vi "Calculate_Deployment_LibInfo.vi"(8 "error in (no error)":errorcluster, 9 "main destination":path, 10 "destinations":refnum<class "AB_Destination.lvclass">[](array[class]), 11 "AB_EXE in":refnum<class "AB_EXE.lvclass">) -> (0 "error out":errorcluster, 2 "Lib Deployment Info":T1, 3 "AB_EXE out":refnum<class "AB_EXE.lvclass">)   [LabVIEW 2020, in "AB_EXE.lvclass"]
uses:
  <vilib>/AppBuilder/AB_Classes/EXE/AB_EXE.lvclass
  <vilib>/AppBuilder/AB_Classes/EXE/AB_EXE.lvclass/AB_EXE.ctl
  <vilib>/AppBuilder/AB_Classes/Build/AB_Build.lvclass
  <vilib>/AppBuilder/AB_Classes/Source/AB_Source.lvclass
  <vilib>/AppBuilder/AB_Classes/Destination/AB_Destination.lvclass
  <vilib>/AppBuilder/Engine/AB_Engine_RTDEP_Dep_Lib_Info.ctl
  <vilib>/AppBuilder/Engine/AB_Engine_RTDEP_LibDeploymentInfo.ctl
  <vilib>/Utility/lvfile.llb/NI_FileType.lvlib
  <vilib>/Utility/lvfile.llb/FT_FileTypes.ctl
  e:/builds/penguin/labview/branches/2020/dev/dist/vi.lib/AppBuilder/AB_Classes/Application/AB_Application.lvclass
  e:/builds/penguin/labview/branches/2020/dev/dist/vi.lib/AppBuilder/AB_Classes/TargetFile/AB_Targetfile.lvclass
  e:/builds/penguin/labview/branches/2020/dev/dist/vi.lib/AppBuilder/AB_Classes/Build/AB_Build.lvclass
  e:/builds/penguin/labview/branches/2020/dev/dist/vi.lib/AppBuilder/AB_Classes/EXE/AB_EXE.lvclass
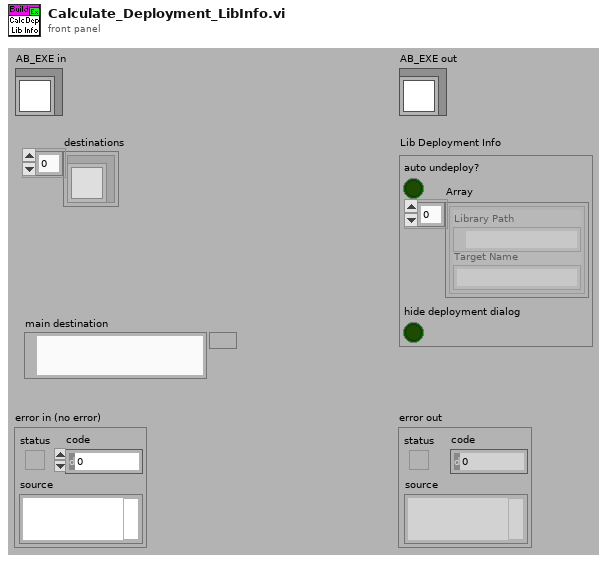
[diagram p1: front panel]
types:
  T1 = typedef "AB_Engine_RTDEP_LibDeploymentInfo.ctl" = cluster{"auto undeploy?":bool, "Array":T2[], "hide deployment dialog":bool}
  T2 = typedef "AB_Engine_RTDEP_Dep_Lib_Info.ctl" = cluster{"Library Path":path, "Target Name":string}
  T3 = typedef "NI_FileType.lvlib/FT_FileTypes.ctl" = enum32{"Invalid file/path", "Unknown type", "Instrument", "Control", "Polymorphic VI", "Project", "Library", "LVClass", "XControl", "XNode", "CIN", "Run-time menu", "Palette menu", "LLB", "Shortcut", "Directory", "Class Private Data Control", "Statechart", "MathScript .m file", "Ladder Diagram", "LVLibp"}
  T4 = typedef "AB_EXE_SharedVar_LibInfo.ctl" = cluster{"LibraryPath":path, "LibraryItemID":string, "target":string, "deploy":bool}
  T5 = typedef "AB_Source.ctl" = cluster{"path":path, "itemID":string, "parentIndex":i32, "sourceInclusion":T6, "destinationIndex":i32, "properties":T7[], "newName":string, "lvfile":bool, "valid":bool, "eng_inBuild":bool, "eng_isNonVILink":bool, "Amalgamation":bool, "Amalgamation Piece":bool, "eng_delimitedName":string, "preventRename":bool}
  T6 = typedef "AB_Source_Inclusion.ctl" = enum16{"IncludeIfReferenced", "Include", "Exclude", "TopLevel"}
  T7 = typedef "AB_Source_Properties.ctl" = cluster{"sourcePropertyType":T8, "value":variant}
  T8 = typedef "AB_Source_Property_Type.ctl" = enum16{"Remove block diagram", "Remove front panel", "Password", "Window has title bar", "Show menu bar", "Show vertical scroll bar", "Show horizontal scroll bar", "Show toolbar", "Show Abort button", "Show fp when called", "Window behavior", "Allow user to close window", "Window run-time position", "Run when opened", "Allow debugging", "Auto error handling", "Generate guard code", "Use stack variables", "Expression folding", "Integer only", "Inline subVI"}
  T9 = typedef "AB_Destination.ctl" = cluster{"destName":string, "path":path, "libraryName":string, "preserveHierarchy":bool, "eng_inBuild":bool, "eng_libraryReference":refnum<vi>, "eng_restictAddToNewLibrary":bool}
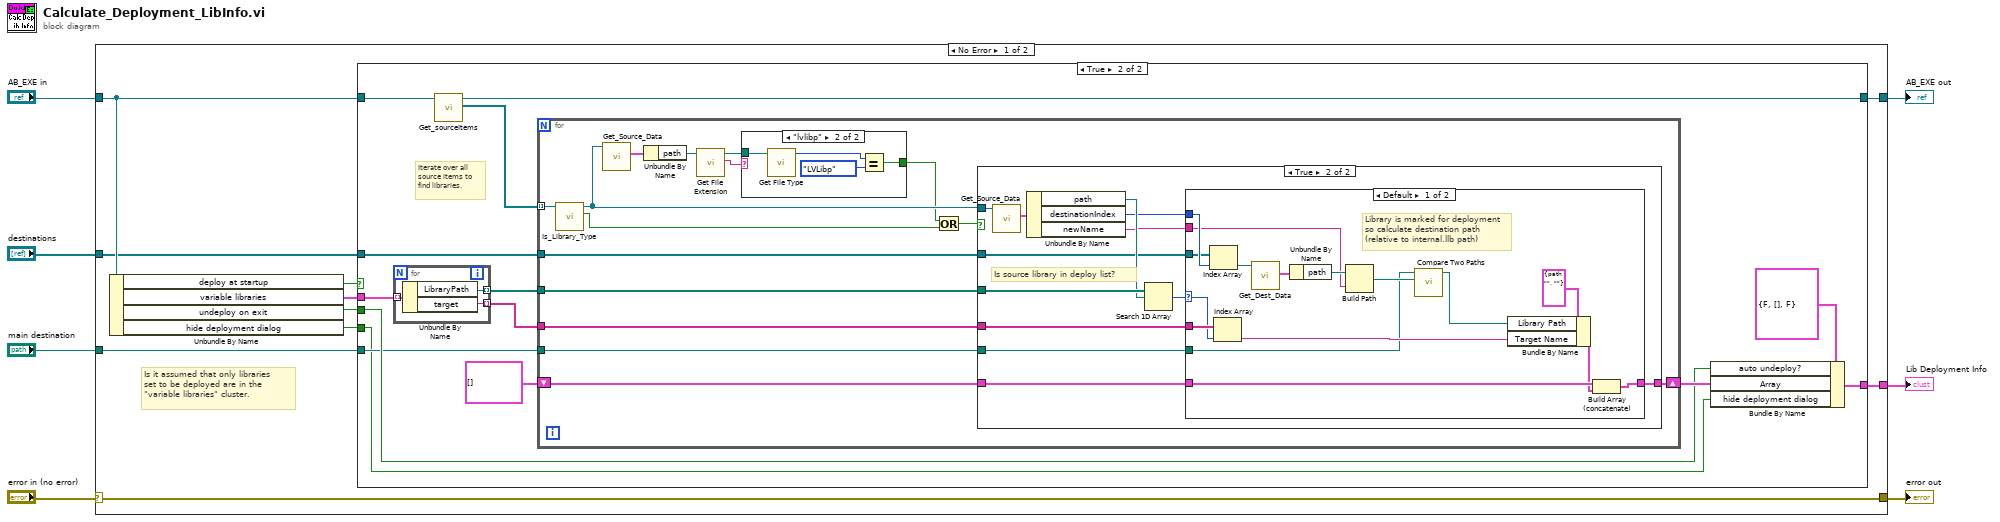
[diagram p0: block diagram]
diagram:
  n1 = case shown="No Error" "error in (no error)" {
    selector: "error in (no error)" -> [w17 w86]
    tunnel: [w17 w86] -> w6
    tunnel: [w14 w85] -> w4
    tunnel: "AB_EXE in" -> [w16 w85]
    tunnel: [w12 _] -> w3
    tunnel: "destinations" -> [w11 _]
    tunnel: "main destination" -> [w10 _]
    frame No Error {
      # "Is it assumed that only libraries set to be deployed are in the \"variable libraries\" cluster."
      n2 = Unbundle By Name(w16) -> ("deploy at startup"=w15:bool, "variable libraries"=w13:T4[], "undeploy on exit"=w9:bool, "hide deployment dialog"=w8:bool)
      n3 = case shown="True" w15 {
        tunnel: w16 -> [w18 w22]
        tunnel: [w18 w32] -> w14
        tunnel: w9 -> [_ w23]
        tunnel: w13 -> [_ w30]
        tunnel: [_ w24] -> w12
        tunnel: w11 -> [_ w21]
        tunnel: w10 -> [_ w20]
        tunnel: w8 -> [_ w19]
        frame False {
        }
        frame True {
          # "Iterate over all source items to find libraries."
          n4 = for {
            tunnel: w30 -> [w35] mode=indexing
            tunnel: [w34] -> w29 mode=indexing
            tunnel: [w33] -> w28 mode=indexing
            n5 = Unbundle By Name(w35) -> ("LibraryPath"=w34:path, "target"=w33:string)
          }
          n6 = call <vilib>:"Get_sourceItems.vi"("Class in"=w22) -> ("sourceItems"=w31:refnum<class "AB_Source.lvclass">[], "Class out"=w32:refnum<class "AB_EXE.lvclass">)  [unwired: 1 in, 8 out]
          n7 = for {
            tunnel: w31 -> [w44] mode=indexing
            tunnel: w29 -> [w50]
            shift-right: [w49] -> w25
            shift-left: T2[] [] -> [w48]
            tunnel: w28 -> [w47]
            tunnel: w21 -> [w46]
            tunnel: w20 -> [w45]
            n8 = call-dynamic "Is_Library_Type.vi"("AB_Source in"=w44) -> ("library type"=w40:bool, "AB_Source out"=w43:refnum<class "AB_Source.lvclass">)  [unwired: 1 in, 8 out]
            n9 = call <vilib>:"Get_Source_Data.vi"("Class in"=w43) -> ("data"=w42:T5)  [unwired: 1 in, 9 out]
            n10 = Unbundle By Name(w42) -> ("path"=w38:path)
            n11 = call <vilib>:"Get File Extension.vi"("file"=w38) -> ("lowercase file extension"=w37:string, "dup file"=w36:path)  [unwired: 6 in, 3 out]
            n12 = case shown="\"lvlibp\"" w37 {
              tunnel: [_ w52] -> w39
              tunnel: w36 -> [_ w51]
              frame Default {
              }
              frame "lvlibp" {
                n13 = call <vilib>:"Get File Type.vi"("path"=w51) -> ("file type"=w54:T3)  [unwired: 8 in, 2 out]
                n14 = Equal?(x=w54, y=FT_FileTypes."LVLibp" ("file type")) -> (x = y?=w52:bool)
              }
            }
            n15 = Or(x=w39, y=w40) -> (x .or. y?=w41:bool)
            n16 = case shown="True" w41 {
              tunnel: w43 -> [_ w56]
              tunnel: w50 -> [_ w67]
              tunnel: [w55 w64] -> w49
              tunnel: w48 -> [w55 w63]
              tunnel: w47 -> [_ w62]
              tunnel: w46 -> [_ w60]
              tunnel: w45 -> [_ w58]
              frame False {
                # "File is not a library so skip."
              }
              frame True {
                # "Is source library in deploy list?"
                n17 = call <vilib>:"Get_Source_Data.vi"("Class in"=w56) -> ("data"=w57:T5)  [unwired: 1 in, 9 out]
                n18 = Unbundle By Name(w57) -> ("path"=w65:path, "destinationIndex"=w61:i32, "newName"=w59:string)
                n19 = Search 1D Array(1D array=w67, element=w65) -> (index of element=w66:i32)  [unwired: 1 out]
                n20 = case shown="Default" w66 {
                  selector: w66 -> [w80 _]
                  tunnel: [w83 w84] -> w64
                  tunnel: w63 -> [w82 w84]
                  tunnel: w62 -> [w81 _]
                  tunnel: w61 -> [w79 _]
                  tunnel: w60 -> [w74 _]
                  tunnel: w59 -> [w75 _]
                  tunnel: w58 -> [w68 _]
                  frame Default {
                    # "Library is marked for deployment so calculate destination path  (relative to internal.llb path)"
                    n21 = Index Array(array=w74, index=w79) -> (element=w78:refnum<class "AB_Destination.lvclass">)
                    n22 = Index Array(array=w81, index=w80) -> (element=w71:string)
                    n23 = call <vilib>:"Get_Dest_Data.vi"("Class in"=w78) -> ("destName"=w77:T9)  [unwired: 1 in, 9 out]
                    n24 = Unbundle By Name(w77) -> ("path"=w76:path)
                    n25 = Build Path(base path=w76, name or relative path=w75) -> (appended path=w73:path)
                    n26 = call <vilib>:"Compare Two Paths.vi"("Path 2"=w73, "Path 1"=w68) -> ("Relative Path from 1 to 2"=w70:path)  [unwired: 1 in, 8 out]
                    n27 = Bundle By Name(cluster=T2 {"Library Path"=path "", "Target Name"=""} ("AB_Engine_RTDEP_Dep_Lib_Info"), "Library Path"=w70, "Target Name"=w71) -> (w69:T2)
                    n28 = Build Array (concatenate)(w82, w69) -> (w83:T2[])
                  }
                  frame -1 {
                  }
                }
              }
            }
          }
          n29 = Bundle By Name(cluster=T1 {"auto undeploy?"=FALSE, "Array"=[], "hide deployment dialog"=FALSE} ("Lib Deployment Info"), "auto undeploy?"=w23, "Array"=w25, "hide deployment dialog"=w19) -> (w24:T1)
        }
      }
    }
    frame Error {
    }
  }
  "error out" <- w6
  "AB_EXE out" <- w4
  "Lib Deployment Info" <- w3
